vi "IO Loop.vi"(7 "Queue in":refnum<queue>, 8 "error in (no error)":errorcluster, 9 "DIO Ref Out":T8, 10 "PWM Ref Out":T1, 11 "PWM Ref Out 2":T1) -> (0 "error out":errorcluster)   [LabVIEW 2015]
uses:
  Controls/RT controls.ctl
  <vilib>/myRIO/Instrument Drivers/Onboard IO/DIO/typedefs/DIO Reference.ctl
  <vilib>/myRIO/Common/Instrument Driver Framework/Utilities/typedefs/myRIO Generic Hardware Reference.ctl
  <vilib>/myRIO/Common/Instrument Driver Framework/Utilities/typedefs/Hardware Version Enum.ctl
  <vilib>/myRIO/Common/Instrument Driver Framework/Utilities/typedefs/myRIO v1.0 Reference.ctl
  <vilib>/myRIO/Common/Instrument Driver Framework/Utilities/typedefs/Generic FPGA Reference.ctl
  <vilib>/myRIO/Common/Instrument Driver Framework/myRIO v1.0/DIO/typedefs/DIO Channels List.ctl
  <vilib>/myRIO/Common/Instrument Driver Framework/myRIO v1.0/DIO/typedefs/DIO Channels Enum.ctl
  <vilib>/myRIO/Instrument Drivers/Onboard IO/PWM/typedefs/PWM Reference.ctl
  <vilib>/myRIO/Common/Instrument Driver Framework/myRIO v1.0/PWM/typedefs/PWM Channels Enum.ctl
  <vilib>/myRIO/Instrument Drivers/Onboard IO/PWM/typedefs/PWM Configuration.ctl
  <vilib>/myRIO/Instrument Drivers/Onboard IO/PWM/vis/Set Duty Cycle and Frequency.vi
  <vilib>/myRIO/Common/Instrument Driver Framework/myRIO v1.0/PWM/vis/myRIO v1.0 Close PWM.vi
  <vilib>/myRIO/Common/Instrument Driver Framework/myRIO v1.0/DIO/vis/myRIO v1.0 Close DIO.vi
  <vilib>/myRIO/Common/Instrument Driver Framework/myRIO v1.0/PWM/vis/myRIO v1.0 Unreserve PWM.vi
  <vilib>/myRIO/Common/Instrument Driver Framework/myRIO v1.0/DIO/vis/myRIO v1.0 Unreserve DIO.vi
  <vilib>/myRIO/Common/Instrument Driver Framework/myRIO v1.0/PWM/vis/myRIO v1.0 Build MUX Configuration PWM.vi
  <vilib>/myRIO/Common/Instrument Driver Framework/myRIO v1.0/Resource Manager/vis/myRIO v1.0 Unreserve Channel List.vi
  <vilib>/myRIO/Common/Instrument Driver Framework/myRIO v1.0/DIO/vis/myRIO v1.0 Build MUX Configuration DIO.vi
  <vilib>/myRIO/Common/Instrument Driver Framework/myRIO v1.0/Resource Manager/vis/myRIO v1.0 Create Configuration List.vi
  <vilib>/myRIO/Common/Instrument Driver Framework/myRIO v1.0/Resource Manager/vis/myRIO v1.0 Unreserve Channel.vi
  <vilib>/myRIO/Common/Instrument Driver Framework/myRIO v1.0/Resource Manager/vis/myRIO v1.0 Build Mutex Name.vi
  <vilib>/Utility/error.llb/Error Cluster From Error Code.vi
  <vilib>/myRIO/Common/Instrument Driver Framework/myRIO v1.0/DIO/vis/myRIO v1.0 Write DIO.vi
  <vilib>/myRIO/Common/Instrument Driver Framework/myRIO v1.0/PWM/vis/myRIO v1.0 Write PWM.vi
  <vilib>/myRIO/Common/Instrument Driver Framework/myRIO v1.0/PWM/vis/myRIO v1.0 Shutdown PWM.vi
  <vilib>/myRIO/Common/Instrument Driver Framework/myRIO v1.0/Resource Manager/vis/myRIO v1.0 Configure IO.vi
  <vilib>/myRIO/Common/Instrument Driver Framework/Utilities/vis/Configuration Manager.vi
  <vilib>/myRIO/Common/Instrument Driver Framework/Utilities/vis/IO Manager.vi
  <vilib>/myRIO/Common/Instrument Driver Framework/myRIO v1.0/myRIO v1.0 Close.vi
  <vilib>/myRIO/Common/Instrument Driver Framework/myRIO v1.0/DIO/vis/myRIO v1.0 Shutdown DIO.vi
  <vilib>/myRIO/Instrument Drivers/Onboard IO/DIO/DIO.lvlib
  <vilib>/myRIO/Instrument Drivers/Onboard IO/PWM/PWM.lvlib
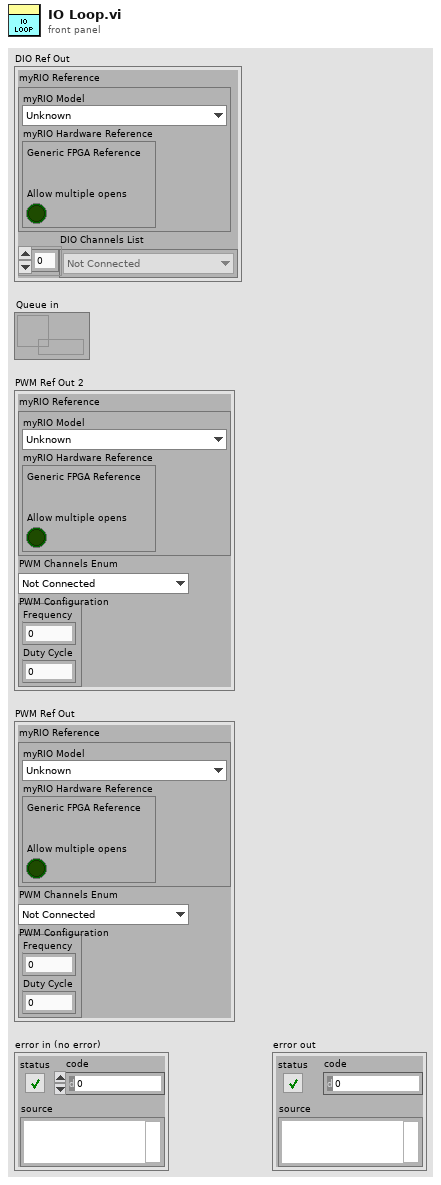
[diagram p1: front panel]
types:
  T1 = typedef "PWM.lvlib/PWM Reference.ctl" = cluster{"myRIO Reference":T2, "PWM Channels Enum":T6, "PWM Configuration":T7}
  T2 = typedef "myRIO Generic Hardware Reference.ctl" = cluster{"myRIO Model":T3, "myRIO Hardware Reference":T4}
  T3 = typedef "Hardware Version Enum.ctl" = enum16{"Unknown", "myRIO-1900", "myRIO-1950", "roboRIO"}
  T4 = typedef "myRIO v1.0 Reference.ctl" = cluster{"Generic FPGA Reference":T5, "Allow multiple opens":bool}
  T5 = typedef "Generic FPGA Reference.ctl" = refnum<k20>
  T6 = typedef "PWM Channels Enum.ctl" = enum16{"Not Connected", "C/PWM0", "C/PWM1", "A/PWM0", "A/PWM1", "A/PWM2", "B/PWM0", "B/PWM1", "B/PWM2", "PWM/PWM0", "PWM/PWM1", "PWM/PWM2", "PWM/PWM3", "PWM/PWM4", "PWM/PWM5", "PWM/PWM6", "PWM/PWM7", "PWM/PWM8", "PWM/PWM9"}
  T7 = typedef "PWM.lvlib/PWM Configuration.ctl" = cluster{"Frequency":dbl, "Duty Cycle":dbl}
  T8 = typedef "DIO.lvlib/DIO Reference.ctl" = cluster{"myRIO Reference":T2, "DIO Channels List":T9}
  T9 = typedef "DIO Channels List.ctl" = T10[]
  T10 = typedef "DIO Channels Enum.ctl" = enum16{"Not Connected", "C/DIO0", "C/DIO1", "C/DIO2", "C/DIO3", "C/DIO4", "C/DIO5", "C/DIO6", "C/DIO7", "A/DIO0", "A/DIO1", "A/DIO2", "A/DIO3", "A/DIO4", "A/DIO5", "A/DIO6", "A/DIO7", "A/DIO8", "A/DIO9", "A/DIO10", "A/DIO11", "A/DIO12", "A/DIO13", "A/DIO14", "A/DIO15", "B/DIO0", "B/DIO1", "B/DIO2", "B/DIO3", "B/DIO4", "B/DIO5", "B/DIO6", "B/DIO7", "B/DIO8", "B/DIO9", "B/DIO10", "B/DIO11", "B/DIO12", "B/DIO13", "B/DIO14", "B/DIO15", "LED0", "LED1", "LED2", "LED3", "Button0", "DIO/DIO0", "DIO/DIO1", "DIO/DIO2", "DIO/DIO3", "DIO/DIO4", "DIO/DIO5", "DIO/DIO6", "DIO/DIO7", "DIO/DIO8", "DIO/DIO9", "SPI/CS0", "SPI/CS1", "SPI/CS2", "SPI/CS3", "LED RADIO (Green)", "LED RADIO (Red)", "LED COMM (Green)", "LED COMM (Red)", "LED MODE (Green)", "LED MODE (Red)"}
  T11 = typedef "RT controls.ctl" = cluster{"PWM width":dbl, "Headlights":bool, "Red Lights":bool, "Left Turn Lights":bool, "Steer Position":dbl, "Right Turn Lights":bool, "Under Lights":bool}
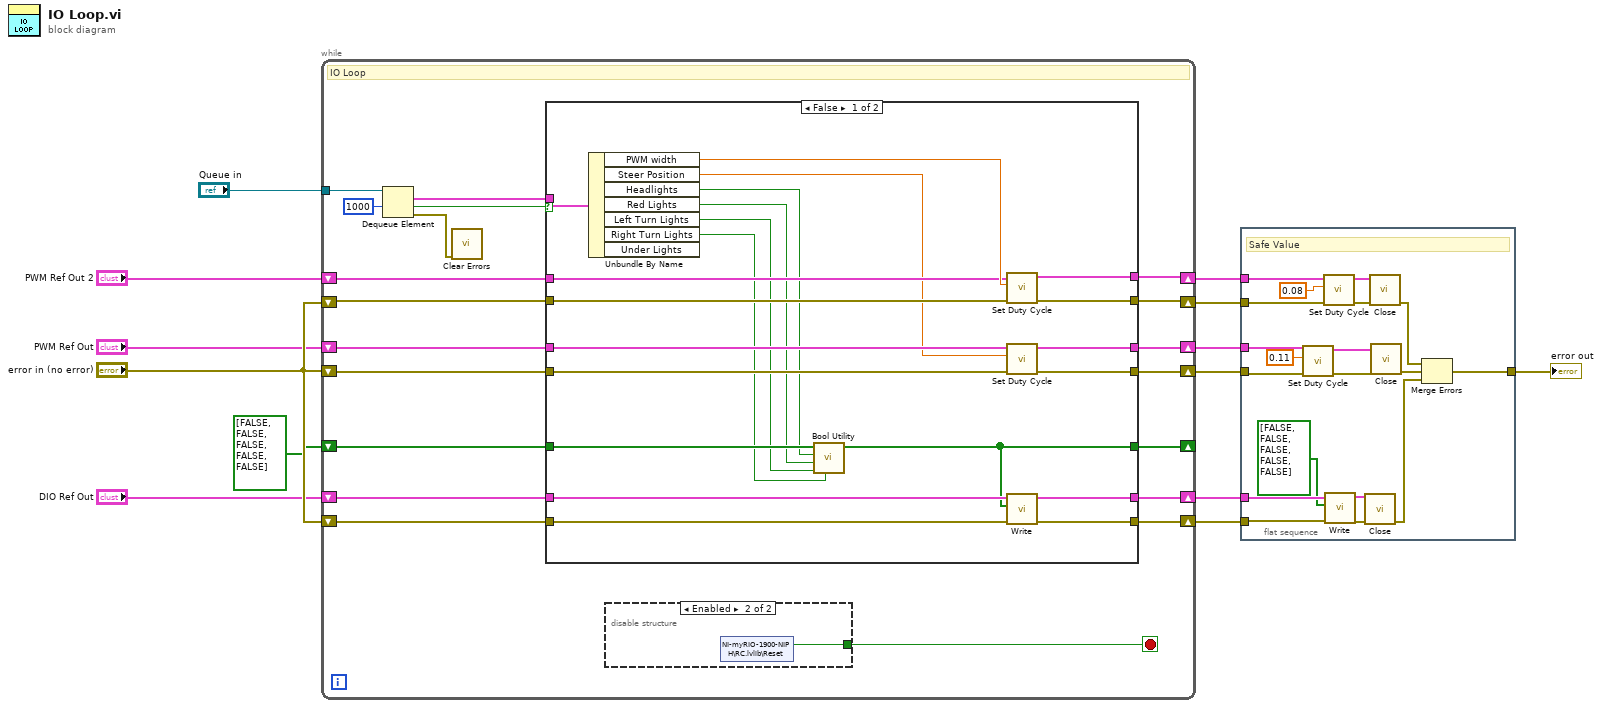
[diagram p0: block diagram]
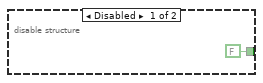
[diagram p2: hidden frame]
diagram:
  n1 = while {
    tunnel: "Queue in" -> [w32]
    shift-right: [w23] -> w8
    shift-left: "PWM Ref Out 2" -> [w27]
    shift-right: [w21] -> w10
    shift-left: "PWM Ref Out" -> [w25]
    shift-right: [w19] -> w6
    shift-left: "DIO Ref Out" -> [w29]
    shift-right: [w20] -> w11
    shift-left: "error in (no error)" -> [w24]
    shift-right: [w22] -> w9
    shift-left: "error in (no error)" -> [w26]
    shift-right: [w18] -> w7
    shift-left: "error in (no error)" -> [w28]
    shift-right: [w16] -> _
    shift-left: bool[] [FALSE, FALSE, FALSE, FALSE, FALSE] ("Values") -> [w17]
    stop <- w14 stop-if-true
    # "IO Loop"
    n2 = Dequeue Element(queue=w32, timeout in ms (-1)=1000) -> (element=w30:T11, timed out?=w31:bool, error out=w15:errorcluster)  [unwired: 1 in, 1 out]
    n3 = call <vilib>:"Clear Errors.vi"("error in (no error)"=w15) -> ()  [unwired: 5 in, 2 out]
    n4 = case shown="False" w31 {
      tunnel: w30 -> [w56 _]
      tunnel: w29 -> [w55 w59]
      tunnel: w28 -> [w54 w58]
      tunnel: w27 -> [w52 w63]
      tunnel: w26 -> [w51 w62]
      tunnel: w25 -> [w50 w61]
      tunnel: w24 -> [w49 w60]
      tunnel: [w48 w63] -> w23
      tunnel: [w47 w62] -> w22
      tunnel: [w46 w61] -> w21
      tunnel: [w45 w60] -> w20
      tunnel: [w44 w59] -> w19
      tunnel: [w43 w58] -> w18
      tunnel: w17 -> [w41 w57]
      tunnel: [w36 w57] -> w16
      frame False {
        n5 = Unbundle By Name(w56) -> ("PWM width"=w53:dbl, "Steer Position"=w42:dbl, "Headlights"=w40:bool, "Red Lights"=w39:bool, "Left Turn Lights"=w38:bool, "Right Turn Lights"=w37:bool)  [unwired: 1 out]
        n6 = call "Bool Utility.vi"("Right Turn Lights"=w37, "Left Turn Lights"=w38, "Red Lights"=w39, "Headlights"=w40, "Values"=w41) -> ("Values Out"=w36:bool[])  [unwired: 6 in]
        n7 = call <vilib>:"Set Duty Cycle.vi"("error in (no error)"=w51, "Duty Cycle"=w53, "PWM Ref In"=w52) -> ("error out"=w47:errorcluster, "PWM Ref Out"=w48:T1)  [unwired: 6 in]
        n8 = call <vilib>:"Set Duty Cycle.vi"("error in (no error)"=w49, "Duty Cycle"=w42, "PWM Ref In"=w50) -> ("error out"=w45:errorcluster, "PWM Ref Out"=w46:T1)  [unwired: 6 in]
        n9 = call <vilib>:"Write.vi"("error in (no error)"=w54, "Values"=w36, "DIO Ref In"=w55) -> ("error out"=w43:errorcluster, "DIO Ref Out"=w44:T8)  [unwired: 6 in]
      }
      frame True {
      }
    }
    n10 = disable-structure shown="Enabled" {
      disable-tunnel: [FALSE w35] -> w14
      frame Disabled {
      }
      frame Enabled {
        n11 = shared-variable "NI-myRIO-1900-NIPH\\RC.lvlib\\Reset"() -> (w35:bool)  [unwired: 1 in, 1 out]
      }
    }
  }
  n12 = flat-sequence {
    tunnel: w6 -> [w77]
    tunnel: w7 -> [w74]
    tunnel: w8 -> [w82]
    tunnel: w9 -> [w81]
    tunnel: w10 -> [w68]
    tunnel: w11 -> [w65]
    tunnel: [w69] -> w13
    frame #0 {
      # "Safe Value"
      n13 = call <vilib>:"Set Duty Cycle.vi"("error in (no error)"=w65, "Duty Cycle"=0.11, "PWM Ref In"=w68) -> ("error out"=w66:errorcluster, "PWM Ref Out"=w67:T1)  [unwired: 6 in]
      n14 = call <vilib>:"Set Duty Cycle.vi"("error in (no error)"=w81, "Duty Cycle"=0.08, "PWM Ref In"=w82) -> ("error out"=w80:errorcluster, "PWM Ref Out"=w78:T1)  [unwired: 6 in]
      n15 = call <vilib>:"Write.vi"("error in (no error)"=w74, "Values"=bool[] [FALSE, FALSE, FALSE, FALSE, FALSE], "DIO Ref In"=w77) -> ("error out"=w75:errorcluster, "DIO Ref Out"=w76:T8)  [unwired: 6 in]
      n16 = call <vilib>:"Close.vi"("error in (no error)"=w75, "DIO Ref In"=w76) -> ("error out"=w70:errorcluster)  [unwired: 9 in]
      n17 = call <vilib>:"Close.vi"("error in (no error)"=w80, "PWM Ref In"=w78) -> ("error out"=w72:errorcluster)  [unwired: 9 in]
      n18 = call <vilib>:"Close.vi"("error in (no error)"=w66, "PWM Ref In"=w67) -> ("error out"=w71:errorcluster)  [unwired: 9 in]
      n19 = Merge Errors(w72, w71, w70) -> (w69:errorcluster)
    }
  }
  "error out" <- w13
